vi "GRNF_DIC.vi"(7 "RefNum Name":string) -> (0 "Error":errorcluster, 3 "Device Reference":T1={"DevStatus"={"status"=FALSE, "code"=0, "source"=""}, "CntIndex"=enum."Invalid"})   [LabVIEW 2019]
doc: "This VI loads an digital input counter refnum on code boot and then stores it in memory so that the information does not have to be queried on subsequent loop cycles. This VI is configured for polymorphic use."
uses:
  <vilib>/Rock Robotics/WPI/Counter/WPI_CounterDevRef.ctl
  <vilib>/Rock Robotics/SystemInterfaces/Counter/FPGA_CounterCtrSystemIndex.ctl
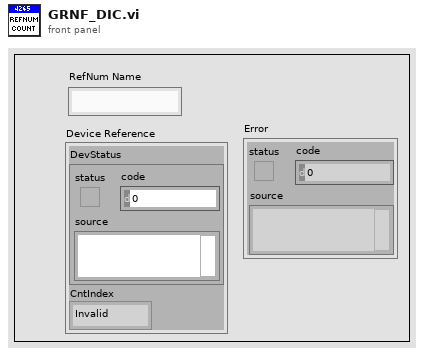
[diagram p1: front panel]
types:
  T1 = typedef "WPI_CounterDevRef.ctl" = cluster{"DevStatus":errorcluster, "CntIndex":T2}
  T2 = typedef "FPGA_CounterCtrSystemIndex.ctl" = enum8{"Ctr 0", "Ctr 1", "Ctr 2", "Ctr 3", "Ctr 4", "Ctr 5", "Ctr 6", "Ctr 7", "Invalid"}
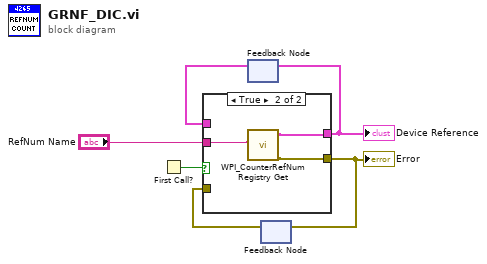
[diagram p0: block diagram]
diagram:
  n1 = First Call?() -> (First Call?: T/F=w6:bool)
  n2 = feedback #1() -> (w5:T1)  [unwired: 1 in]
  n3 = feedback #2() -> (w1:errorcluster)  [unwired: 1 in]
  n4 = case shown="True" w6 {
    tunnel: [w8 w11] -> w4
    tunnel: w5 -> [w8 _]
    tunnel: "RefNum Name" -> [_ w9]
    tunnel: [w7 w10] -> w2
    tunnel: w1 -> [w7 _]
    frame False {
    }
    frame True {
      n5 = call <vilib>:"WPI_CounterRefNum Registry Get.vi"("refnum name"=w9) -> ("error out"=w10:errorcluster, "CounterDevRef"=w11:T1)  [unwired: 9 in]
    }
  }
  "Error" <- w2
  "Device Reference" <- w4
  n6 = feedback-in #1(w4) -> ()
  n7 = feedback-in #2(w2) -> ()
